vi "Telescope Move to RA and DEC.vi"(8 "error in (no error)":errorcluster, 9 "Offset?":bool, 10 "Object in":T1, 11 "LDT Telescope in":refnum<class "LDT Telescope.lvclass">) -> (0 "error out":errorcluster, 3 "LDT Telescope out":refnum<class "LDT Telescope.lvclass">)   [LabVIEW 2022 SP3, in "LDT Telescope.lvclass"]
uses:
  LDT Telescope.lvclass
  typedefs/CC cluster Object.ctl
  typedefs/CC cluster sidereal rate.ctl
  typedefs/CC cluster RA and DEC.ctl
  typedefs/cc cluster muRA muDEC.ctl
  CC cluster Telescope Offsets.ctl
  Telescope cluster Equinox.ctl
  Telescope cluster Parallax.ctl
  Telescope cluster Rotator.ctl
  Telesope ring Frame.ctl
  LDT Telescope.lvclass/LDT Telescope.ctl
  Telescope.lvclass
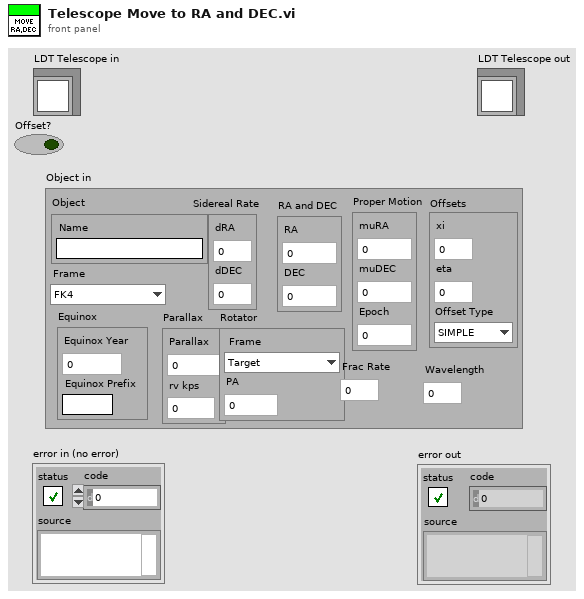
[diagram p1: front panel]
types:
  T1 = typedef "CC cluster Object.ctl" = cluster{"Object":cluster{"Name":string}, "Sidereal Rate":T2, "RA and DEC":T3, "Proper Motion":T4, "Offsets":T5, "Equinox":T6, "Parallax":T7, "Rotator":T8, "Frame":T9, "Frac Rate":dbl, "Wavelength":dbl}
  T2 = typedef "CC cluster sidereal rate.ctl" = cluster{"dRA":dbl, "dDEC":dbl}
  T3 = typedef "CC cluster RA and DEC.ctl" = cluster{"RA":dbl, "DEC":dbl}
  T4 = typedef "cc cluster muRA muDEC.ctl" = cluster{"muRA":dbl, "muDEC":dbl, "Epoch":dbl}
  T5 = typedef "CC cluster Telescope Offsets.ctl" = cluster{"xi":dbl, "eta":dbl, "Offset Type":enum16{"SIMPLE", "TPLANE", "PA"}}
  T6 = typedef "Telescope cluster Equinox.ctl" = cluster{"Equinox Year":i32, "Equinox Prefix":string}
  T7 = typedef "Telescope cluster Parallax.ctl" = cluster{"Parallax":dbl, "rv kps":dbl}
  T8 = typedef "Telescope cluster Rotator.ctl" = cluster{"Frame":enum16{"Target", "Fixed"}, "PA":dbl}
  T9 = typedef "Telesope ring Frame.ctl" = enum16{"FK4", "FK5", "APPT", "GAPPT", "AZEL"}
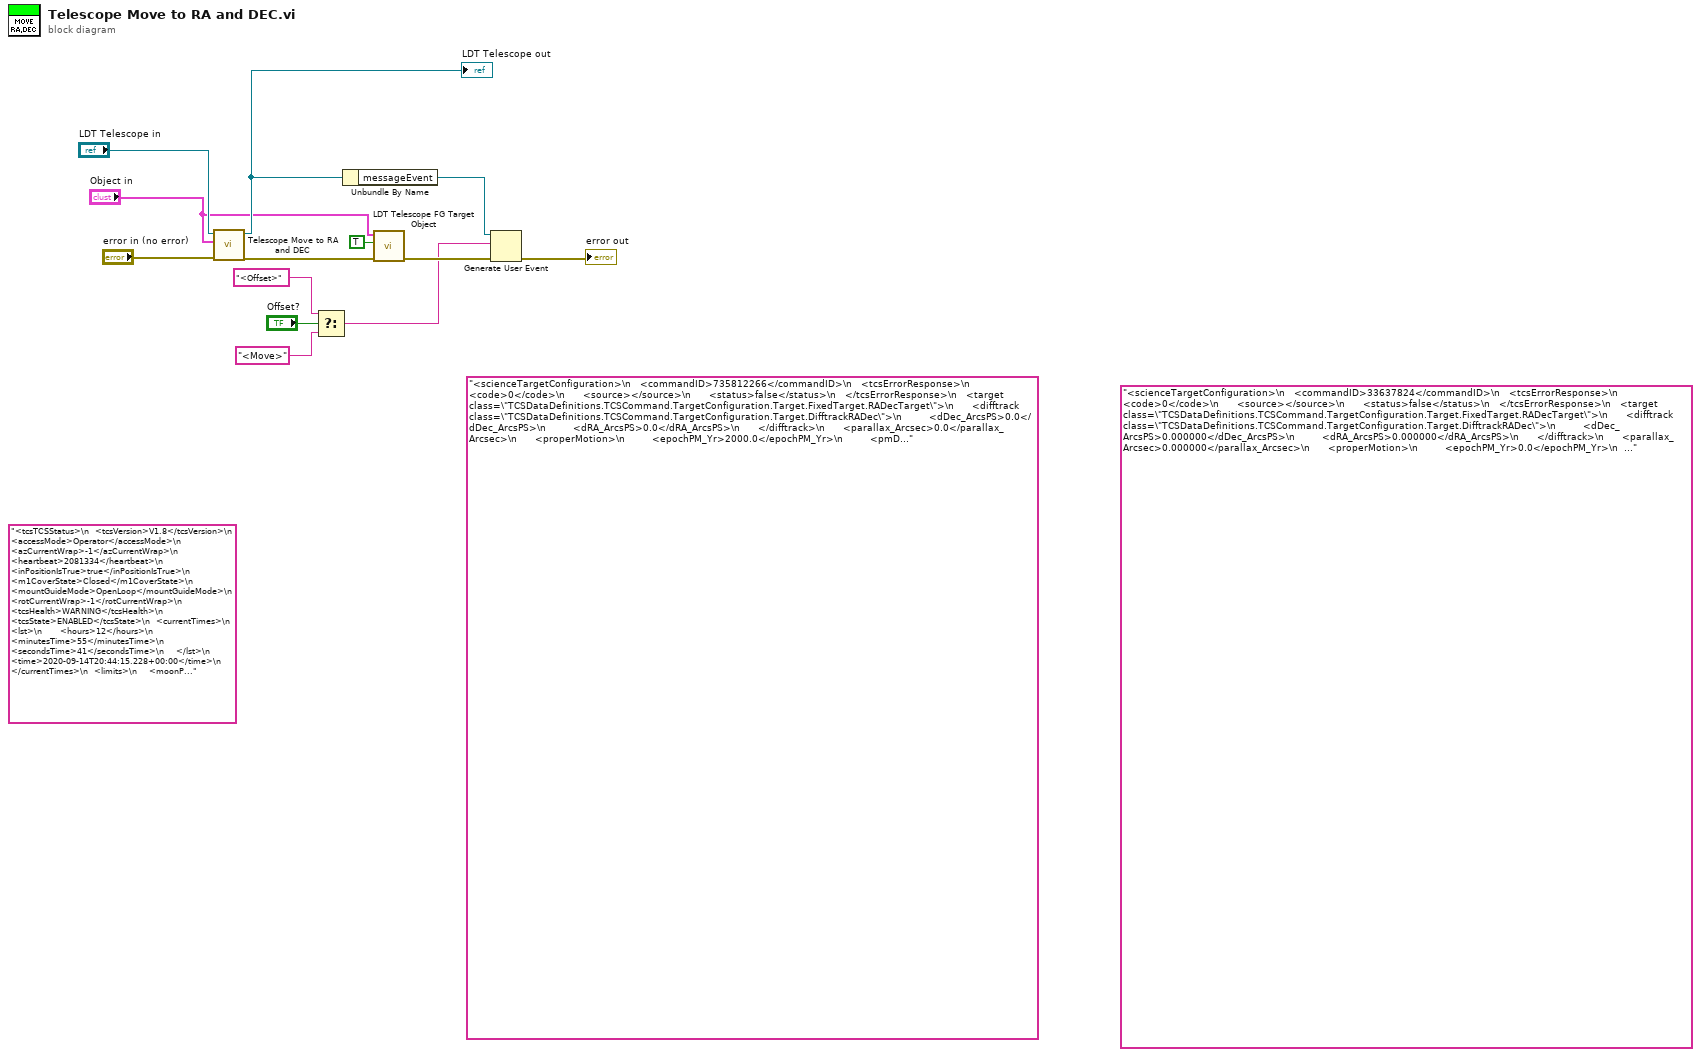
[diagram p0: block diagram]
diagram:
  (unwired) "<scienceTargetConfiguration>\n   <commandID>33637824</commandID>\n   <tcsErrorResponse>\n      <code>0</code>\n      <source></source>\n      <status>false</status>\n   </tcsErrorResponse>\n   <target class=\"TCSDataDefinitions.TCSCommand.TargetConfiguration.Target.FixedTarget.RADecTarget\">\n      <difftrack class=\"TCSDataDefinitions.TCSCommand.TargetConfiguration.Target.DifftrackRADec\">\n         <dDec_ArcsPS>0.000000</dDec_ArcsPS>\n         <dRA_ArcsPS>0.000000</dRA_ArcsPS>\n      </difftrack>\n      <parallax_Arcsec>0.000000</parallax_Arcsec>\n      <properMotion>\n         <epochPM_Yr>0.0</epochPM_Yr>\n         <pmDec_masPYr>0.000000</pmDec_masPYr>\n         <pmRA_masPYr>0.000000</pmRA_masPYr>\n      </properMotion>\n      <rv_kps>0.000000</rv_kps>\n      <targetName>Object111</targetName>\n      <raDecParameters>\n         <declination>\n            <degreesDec>69.000000</degreesDec>\n            <minutesArc>0.0</minutesArc>\n            <secondsArc>0.4</secondsArc>\n         </declination>\n         <equinoxPrefix>J</equinoxPrefix>\n         <equinoxYear>2000.0</equinoxYear>\n         <frame>1</frame>\n         <ra>\n            <hours>8.000000</hours>\n            <minutesTime>20.0</minutesTime>\n            <secondsTime>0.2</secondsTime>\n         </ra>\n      </raDecParameters>\n   </target>\n   <targetConfigName>Object111</targetConfigName>\n   <wl_microns>0.500000</wl_microns>\n   <fracrate>1.000000</fracrate>\n   <rotator>\n      <rotPA>0.000000</rotPA>\n      <rotatorFrame>Target</rotatorFrame>\n   </rotator>\n</scienceTargetConfiguration>"
  (unwired) "<scienceTargetConfiguration>\n   <commandID>735812266</commandID>\n   <tcsErrorResponse>\n      <code>0</code>\n      <source></source>\n      <status>false</status>\n   </tcsErrorResponse>\n   <target class=\"TCSDataDefinitions.TCSCommand.TargetConfiguration.Target.FixedTarget.RADecTarget\">\n      <difftrack class=\"TCSDataDefinitions.TCSCommand.TargetConfiguration.Target.DifftrackRADec\">\n         <dDec_ArcsPS>0.0</dDec_ArcsPS>\n         <dRA_ArcsPS>0.0</dRA_ArcsPS>\n      </difftrack>\n      <parallax_Arcsec>0.0</parallax_Arcsec>\n      <properMotion>\n         <epochPM_Yr>2000.0</epochPM_Yr>\n         <pmDec_masPYr>12.5</pmDec_masPYr>\n         <pmRA_masPYr>7.0</pmRA_masPYr>\n      </properMotion>\n      <rv_kps>0.0</rv_kps>\n      <targetName>TYC 4782-00940-1</targetName>\n      <raDecParameters>\n         <declination>\n            <degreesDec>-0.3200583333333333</degreesDec>\n            <minutesArc>0.0</minutesArc>\n            <secondsArc>0.0</secondsArc>\n         </declination>\n         <equinoxPrefix>J</equinoxPrefix>\n         <equinoxYear>2000.0</equinoxYear>\n         <frame>FK5</frame>\n         <ra>\n            <hours>6.001030833333333</hours>\n            <minutesTime>0.0</minutesTime>\n            <secondsTime>0.0</secondsTime>\n         </ra>\n      </raDecParameters>\n   </target>\n   <targetConfigName>TYC 4782-00940-1</targetConfigName>\n   <wl_microns>0.5</wl_microns>\n   <fracrate>1.0</fracrate>\n   <rotator>\n      <rotPA>0.0</rotPA>\n      <rotatorFrame>Target</rotatorFrame>\n   </rotator>\n</scienceTargetConfiguration>"
  (unwired) "<tcsTCSStatus>\n  <tcsVersion>V1.8</tcsVersion>\n  <accessMode>Operator</accessMode>\n  <azCurrentWrap>-1</azCurrentWrap>\n  <heartbeat>2081334</heartbeat>\n  <inPositionIsTrue>true</inPositionIsTrue>\n  <m1CoverState>Closed</m1CoverState>\n  <mountGuideMode>OpenLoop</mountGuideMode>\n  <rotCurrentWrap>-1</rotCurrentWrap>\n  <tcsHealth>WARNING</tcsHealth>\n  <tcsState>ENABLED</tcsState>\n  <currentTimes>\n    <lst>\n      <hours>12</hours>\n      <minutesTime>55</minutesTime>\n      <secondsTime>41</secondsTime>\n    </lst>\n    <time>2020-09-14T20:44:15.228+00:00</time>\n  </currentTimes>\n  <limits>\n    <moonProximity>\n      <distance_deg>51.647106572866</distance_deg>\n      <proximityFlag>false</proximityFlag>\n    </moonProximity>\n    <sunProximity>\n      <distance_deg>16.531164188648</distance_deg>\n      <proximityFlag>false</proximityFlag>\n    </sunProximity>\n    <zenith>\n      <currentZD_deg>46.221286</currentZD_deg>\n      <elZenithLimit_deg>89.3</elZenithLimit_deg>\n      <inBlindSpotIsTrue>false</inBlindSpotIsTrue>\n      <timeToBlindSpot_min>-1</timeToBlindSpot_min>\n      <timeToBlindSpotExit_min>-1</timeToBlindSpotExit_min>\n    </zenith>\n    <airmass>1.4438282807451</airmass>\n    <currentTimeToObservable_min>-1</currentTimeToObservable_min>\n    <currentTimeToUnobservable_min>262</currentTimeToUnobservable_min>\n    <timeToRotLimit_min>-1</timeToRotLimit_min>\n    <timeToAzLimit_min>-1</timeToAzLimit_min>\n  </limits>\n  <pointingPositions>\n    <azElError>\n      <azError>-0.9792</azError>\n      <elError>0.1584</elError>\n    </azElError>\n    <currentAzEl>\n      <azimuth>\n        <degreesArc>194</degreesArc>\n        <minutesArc>45</minutesArc>\n        <secondsArc>0.7</secondsArc>\n      </azimuth>\n      <elevation>\n        <degreesAlt>43</degreesAlt>\n        <minutesArc>46</minutesArc>\n        <secondsArc>43.4</secondsArc>\n      </elevation>\n    </currentAzEl>\n    <currentHA>\n      <hours>0</hours>\n      <minutesTime>44</minutesTime>\n      <secondsTime>2.04</secondsTime>\n    </currentHA>\n    <currentRADec>\n      <declination>\n        <degreesDec>-10</degreesDec>\n        <minutesArc>15</minutesArc>\n        <secondsArc>25</secondsArc>\n      </declination>\n      <equinoxPrefix>J</equinoxPrefix>\n      <equinoxYear>2000</equinoxYear>\n      <frame>FK5</frame>\n      <ra>\n        <hours>12</hours>\n        <minutesTime>10</minutesTime>\n        <secondsTime>35.34</secondsTime>\n      </ra>\n    </currentRADec>\n    <currentParAngle>12.557342470137</currentParAngle>\n    <currentRotatorPositions>\n      <rotPA>342.260103</rotPA>\n      <iaa>185.2</iaa>\n      <rotIPA>0</rotIPA>\n    </currentRotatorPositions>\n    <difftrackStatus>\n      <dAz_ArcsPS>0</dAz_ArcsPS>\n      <dEl_ArcsPS>0</dEl_ArcsPS>\n      <dRA_ArcsPS>0</dRA_ArcsPS>\n      <dDec_ArcsPS>0</dDec_ArcsPS>\n    </difftrackStatus>\n    <objectPA>\n      <EqPA>-0</EqPA>\n      <AzPA>12.557342470137</AzPA>\n    </objectPA>\n    <demandAzEl>\n      <azimuth>\n        <degreesArc>194</degreesArc>\n        <minutesArc>45</minutesArc>\n        <secondsArc>3.68</secondsArc>\n      </azimuth>\n      <elevation>\n        <degreesAlt>43</degreesAlt>\n        <minutesArc>46</minutesArc>\n        <secondsArc>42.89</secondsArc>\n      </elevation>\n    </demandAzEl>\n    <demandRADec>\n      <declination>\n        <degreesDec>-10</degreesDec>\n        <minutesArc>15</minutesArc>\n        <secondsArc>25</secondsArc>\n      </declination>\n      <equinoxPrefix>J</equinoxPrefix>\n      <equinoxYear>2000</equinoxYear>\n      <frame>FK5</frame>\n      <ra>\n        <hours>12</hours>\n        <minutesTime>10</minutesTime>\n        <secondsTime>35.24</secondsTime>\n      </ra>\n    </demandRADec>\n    <demandRotatorPositions>\n      <rotPA>342.259442</rotPA>\n    </demandRotatorPositions>\n    <targetName>unspecified</targetName>\n  </pointingPositions>\n  <OffsetStatus>\n    <offsetType>SIMPLE</offsetType>\n    <userOff1>0</userOff1>\n    <userOff2>0</userOff2>\n    <handsetOff1>0</handsetOff1>\n    <handsetOff2>0</handsetOff2>\n  </OffsetStatus>\n  <axesTrackMode>All</axesTrackMode>\n  <inPositionAzIsTrue>true</inPositionAzIsTrue>\n  <inPositionElIsTrue>true</inPositionElIsTrue>\n  <inPositionRotIsTrue>true</inPositionRotIsTrue>\n  <externalTargetCfgCmdPreviewIsTrue>true</externalTargetCfgCmdPreviewIsTrue>\n</tcsTCSStatus>"
  n1 = call-parent "Telescope Move to RA and DEC.vi"("error in (no error)"="error in (no error)", "Object out"="Object in", "Telescope in"="LDT Telescope in") -> ("error out"=w10:errorcluster, "Telescope out"=w11:refnum<class "LDT Telescope.lvclass">)  [unwired: 7 in]
  "LDT Telescope out" <- w11
  n2 = Select(t="<Offset>" ("event data"), s="Offset?", f="<Move>" ("event data")) -> (s? t:f=w1:string)
  n3 = Unbundle By Name(w11) -> ("messageEvent"=w6:refnum<user-event>)
  n4 = call "LDT Telescope FG Target Object.vi"("error in (no error)"=w10, "Write?"=TRUE, "Object"="Object in") -> ("error out"=w7:errorcluster)  [unwired: 7 in, 1 out]
  n5 = Generate User Event(user event=w6, event data cluster=w1, error in=w7) -> (error out=→"error out":errorcluster)  [unwired: 1 in, 1 out]
